vi "Write size.vi"(10 "Size":u32, 11 "ITem":refnum<class "file_Item.lvclass">) -> (3 "ITem In Out":refnum<class "file_Item.lvclass">)   [LabVIEW 2020, in "file_Item.lvclass"]
uses:
  file_Item.lvclass
  file_Item.lvclass/file_Item.ctl
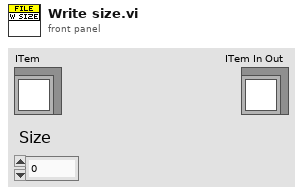
[diagram p1: front panel]
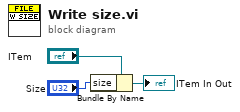
[diagram p0: block diagram]
diagram:
  n1 = Bundle By Name(cluster="ITem", "size"="Size") -> (→"ITem In Out":refnum<class "file_Item.lvclass">)
